vi "Distribute.vi"(8 "error in (no error)":errorcluster, 10 "Bounds":T1, 11 "Container in":refnum<class "Interaction.lvclass">) -> (0 "error out":errorcluster, 2 "Bounds":T1[](array[typedef]), 3 "Container out":refnum<class "Interaction.lvclass">, 5 "Visible bounds":T1[](array[typedef]), 7 "Visible indices":i32[](array[numeric]))   [LabVIEW 2013, in "Interaction.lvclass"]
doc: "Copyright 2018, Wiebe Walstra, wiebe@carya.nl."
uses:
  Interaction.lvclass
  <vilib>/Utility/miscctls.llb/LVRectTypeDef.ctl
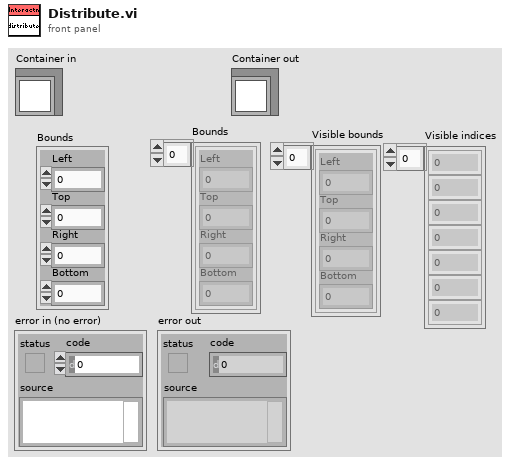
[diagram p1: front panel]
types:
  T1 = typedef "LVRectTypeDef.ctl" = cluster{"Left":i16, "Top":i16, "Right":i16, "Bottom":i16}
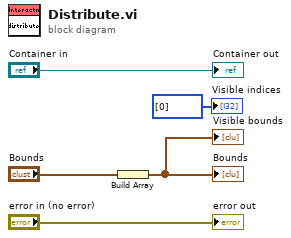
[diagram p0: block diagram]
diagram:
  n1 = Build Array("Bounds") -> (→"Bounds" →"Visible bounds":T1[])
  "error out" <- "error in (no error)"
  "Container out" <- "Container in"
  "Visible indices" <- i32[] [0] ("Visible indices")
